vi "uStringManipulation_replacePrefix_Set.vi"(8 "error in (no error)":errorcluster, 9 "to":string, 10 "from":string, 11 "replacePrefix in":refnum<class "replacePrefix.lvclass">) -> (0 "error out":errorcluster, 3 "replacePrefix out":refnum<class "replacePrefix.lvclass">)   [LabVIEW 2023, in "uLib.lvlib" / "replacePrefix.lvclass"]
doc: "Set the substring replacement. The prefix 'from' substring is replaced with the 'to'."
uses:
  replacePrefix.lvclass
  replacePrefix.lvclass/replacePrefix.ctl
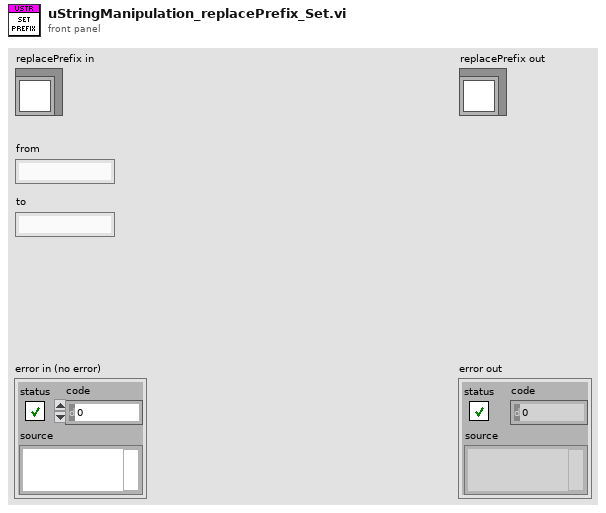
[diagram p1: front panel]
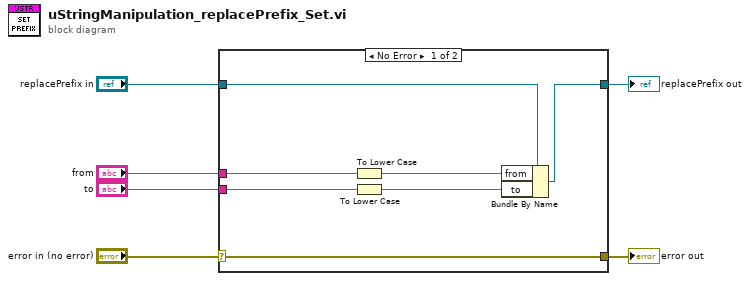
[diagram p0: block diagram]
diagram:
  n1 = case shown="No Error" "error in (no error)" {
    selector: "error in (no error)" -> [w13 w14]
    tunnel: [w13 w14] -> w5
    tunnel: [w11 w15] -> w3
    tunnel: "replacePrefix in" -> [w12 w15]
    tunnel: "from" -> [w10 _]
    tunnel: "to" -> [w8 _]
    frame No Error {
      n2 = To Lower Case(string=w10) -> (all lower case string=w9:string)
      n3 = To Lower Case(string=w8) -> (all lower case string=w7:string)
      n4 = Bundle By Name(cluster=w12, "from"=w9, "to"=w7) -> (w11:refnum<class "replacePrefix.lvclass">)
    }
    frame Error {
    }
  }
  "error out" <- w5
  "replacePrefix out" <- w3
